vi "OP600ZP_CLUSTER_OCVACIR.vi"(10 "MESURES_OCV":cluster{string, string}, 11 "Tableau 3":string[][](array[string])) -> (2 "Tableau":bool[](array[boolean]), 3 "Tableau 2":string[][](array[string]))   [LabVIEW 2020]
uses:
  VG/Ubatt.vi
  OP600ZP_VGConf.vi
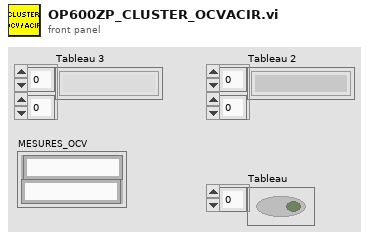
[diagram p1: front panel]
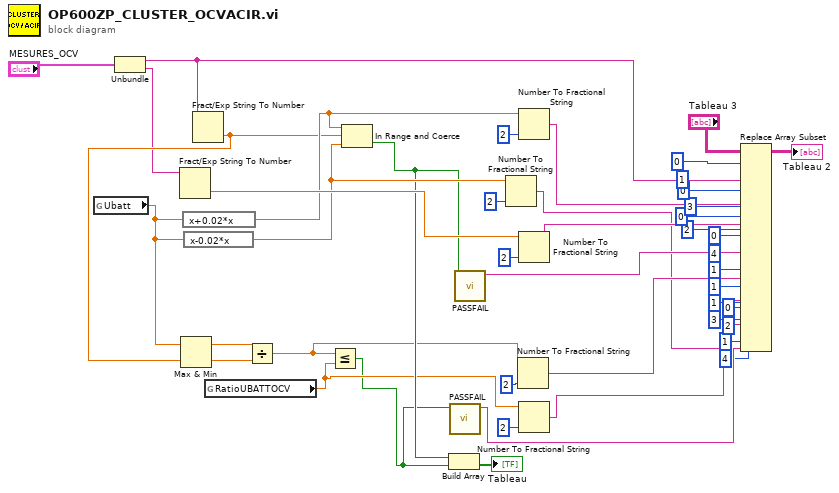
[diagram p0: block diagram]
diagram:
  n1 = global read "Ubatt.vi" "Ubatt"() -> (w30:dbl)
  n2 = Unbundle("MESURES_OCV") -> (w29:string, w7:string)
  n3 = Fract/Exp String To Number(string=w7) -> (number=w42:dbl)  [unwired: 3 in, 1 out]
  n4 = expression code="x+0.02*x"(w30) -> (w39:dbl)
  n5 = expression code="x-0.02*x"(w30) -> (w40:dbl)
  n6 = Fract/Exp String To Number(string=w29) -> (number=w31:dbl)  [unwired: 3 in, 1 out]
  n7 = Max & Min(x=w30, y=w31) -> (max(x,y)=w33:dbl, min(x,y)=w32:dbl)
  n8 = global read "OP600ZP_VGConf.vi" "RatioUBATTOCV"() -> (w12:dbl)
  n9 = Divide(x=w33, y=w32) -> (x/y=w17:dbl)
  n10 = Less Or Equal?(x=w17, y=w12) -> (x <= y?=w8:bool)
  n11 = In Range and Coerce(upper limit=w39, x=w31, lower limit=w40) -> (In Range?=w38:bool)  [unwired: 1 out]
  n12 = Build Array(w38, w8) -> (→"Tableau":bool[])
  n13 = call <userlib>:"PASSFAIL.vi"("E"=w8) -> ("S"=w3:string)  [unwired: 10 in]
  n14 = call <userlib>:"PASSFAIL.vi"("E"=w38) -> ("S"=w20:string)  [unwired: 10 in]
  n15 = Number To Fractional String(number=w40, precision (6)=i16 2 ("précision (6)")) -> (F-format string=w6:string)  [unwired: 2 in]
  n16 = Number To Fractional String(number=w17, precision (6)=i16 2 ("précision (6)")) -> (F-format string=w16:string)  [unwired: 2 in]
  n17 = Number To Fractional String(number=w39, precision (6)=i16 2 ("précision (6)")) -> (F-format string=w26:string)  [unwired: 2 in]
  n18 = Number To Fractional String(number=w42, precision (6)=i16 2 ("précision (6)")) -> (F-format string=w25:string)  [unwired: 2 in]
  n19 = Number To Fractional String(number=w12, precision (6)=i16 2 ("précision (6)")) -> (F-format string=w11:string)  [unwired: 2 in]
  n20 = Replace Array Subset(array="Tableau 3", new element #1=w29, index (row) #1=0 ("indice (ligne)"), index (col) #1=1 ("indice désactivé (col)"), new element #2=w26, index (row) #2=0 ("indice (ligne)"), index (col) #2=3 ("indice désactivé (col)"), new element #3=w25, index (row) #3=0 ("indice (ligne)"), index (col) #3=2 ("indice désactivé (col)"), new element #4=w20, index (row) #4=0 ("indice (ligne)"), index (col) #4=4 ("indice désactivé (col)"), new element #5=w16, index (row) #5=1 ("indice (ligne)"), index (col) #5=1 ("indice désactivé (col)"), new element #6=w11, index (row) #6=1 ("indice (ligne)"), index (col) #6=3 ("indice désactivé (col)"), new element #7=w6, index (row) #7=0 ("indice (ligne)"), index (col) #7=2 ("indice désactivé (col)"), new element #8=w3, index (row) #8=1 ("indice (ligne)"), index (col) #8=4 ("indice désactivé (col)")) -> (→"Tableau 2":string[][])
